vi "TurnScanParabolic2Components.vi"(0 "Start [s] AD raster":dbl=0.000225, 1 "TurnParameters":T1={"Turntime [s]"=4.500000000000001e-05, "Galvo cycle"=1e-05, "Pixeltime"=2.25e-06}, 2 "deltaPosition [m]":cluster{"x":dbl, "y":dbl}={"x"=-4.992779683200315e-05, "y"=-1.09458111857715e-05}, 4 "xPixel":i32=-99, 5 "speed [m/s]":cluster{"x":dbl, "y":dbl}={"x"=0.21752211986383552, "y"=0.04546254963512117}) -> (6 "Ende [s] AD+g raster":dbl=0.00027, 8 "ScanSteuerung":T2(array[cluster])=[{"Zeitpunkt [s]"=0.000225, "Wirkung"=enum."Inc", "Kanal"=enum."Image1X", "Wert (/s)"=-2315789.47368421}, {"Zeitpunkt [s]"=0.000225, "Wirkung"=enum."Rel", "Kanal"=enum."Image1Y", "Wert (/s)"=1.0}, {"Zeitpunkt [s]"=0.00023, "Wirkung"=enum."Abs", "Kanal"=enum."Digital", "Wert (/s)"=5.0}, {"Zeitpunkt [s]"=0.00023, "Wirkung"=enum."IncInc", "Kanal"=enum."GalvoX", "Wert (/s)"=-146143.4081327828}, {"Zeitpunkt [s]"=0.00023, "Wirkung"=enum."IncInc", "Kanal"=enum."GalvoY", "Wert (/s)"=-32321.565855881716}, {"Zeitpunkt [s]"=0.00025, "Wirkung"=enum."IncInc", "Kanal"=enum."GalvoX", "Wert (/s)"=146143.4081327828}, {"Zeitpunkt [s]"=0.00025, "Wirkung"=enum."IncInc", "Kanal"=enum."GalvoY", "Wert (/s)"=32321.565855881716}, {"Zeitpunkt [s]"=0.00026775000000000003, "Wirkung"=enum."Inc", "Kanal"=enum."Image1X", "Wert (/s)"=0.0}, {"Zeitpunkt [s]"=0.00027, "Wirkung"=enum."Abs", "Kanal"=enum."Digital", "Wert (/s)"=7.0}])   [LabVIEW 2011]
panel:
  out "t1":dbl=2e-05
  out "t0":dbl=2e-05
  out "x-y*floor(x/y)==galvoToo late":dbl=5.000000000000006e-06
  out "available galvo cycles":dbl=4.0
  # "For unidirectional!"
  # "ImageX is stopped before\ngalvos are still moving!"
  # "ImageX is stopped before\ngalvos are still moving!"
  # "Trigger Start Turn :101\nTrigger End Turn: 111"
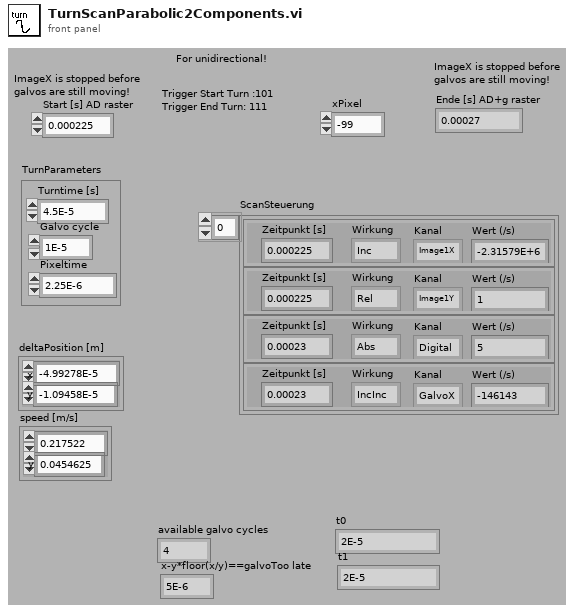
[diagram p1: front panel]
types:
  T1 = cluster{"Turntime [s]":dbl, "Galvo cycle":dbl, "Pixeltime":dbl}
  T2 = cluster{"Zeitpunkt [s]":dbl, "Wirkung":enum16{"Abs", "Rel", "Inc", "IncInc", "LoopStart", "LoopEnd"}, "Kanal":enum16{"Com", "AnalogConfig", "AnalogValue", "GalvoX", "GalvoY", "Galvo3", "Galvo4", "Digital", "Free", "Loop", "SMoveTime", "Image1X", "Image1Y", "Image2X", "Image2Y"}, "Wert (/s)":dbl}[]
  T3 = enum16{"Com", "AnalogConfig", "AnalogValue", "GalvoX", "GalvoY", "Galvo3", "Galvo4", "Digital", "Free", "Loop", "SMoveTime", "Image1X", "Image1Y", "Image2X", "Image2Y"}
  T4 = enum16{"Abs", "Rel", "Inc", "IncInc", "LoopStart", "LoopEnd"}
  T5 = cluster{"Start [s] AD raster":dbl, "Wirkung":enum16{"Abs", "Rel", "Inc", "IncInc", "LoopStart", "LoopEnd"}, "Kanal":enum16{"Com", "AnalogConfig", "AnalogValue", "GalvoX", "GalvoY", "Galvo3", "Galvo4", "Digital", "Free", "Loop", "SMoveTime", "Image1X", "Image1Y", "Image2X", "Image2Y"}, dbl}
  T6 = cluster{dbl, "Wirkung":enum16{"Abs", "Rel", "Inc", "IncInc", "LoopStart", "LoopEnd"}, "Kanal":enum16{"Com", "AnalogConfig", "AnalogValue", "GalvoX", "GalvoY", "Galvo3", "Galvo4", "Digital", "Free", "Loop", "SMoveTime", "Image1X", "Image1Y", "Image2X", "Image2Y"}, "y":dbl}
  T7 = cluster{dbl, "Wirkung":enum16{"Abs", "Rel", "Inc", "IncInc", "LoopStart", "LoopEnd"}, "Kanal":enum16{"Com", "AnalogConfig", "AnalogValue", "GalvoX", "GalvoY", "Galvo3", "Galvo4", "Digital", "Free", "Loop", "SMoveTime", "Image1X", "Image1Y", "Image2X", "Image2Y"}, "x":dbl}
  T8 = cluster{dbl, "Wirkung":enum16{"Abs", "Rel", "Inc", "IncInc", "LoopStart", "LoopEnd"}, "Kanal":enum16{"Com", "AnalogConfig", "AnalogValue", "GalvoX", "GalvoY", "Galvo3", "Galvo4", "Digital", "Free", "Loop", "SMoveTime", "Image1X", "Image1Y", "Image2X", "Image2Y"}, u8}
  T9 = cluster{"Start [s] AD raster":dbl, "Wirkung":enum16{"Abs", "Rel", "Inc", "IncInc", "LoopStart", "LoopEnd"}, "Kanal":enum16{"Com", "AnalogConfig", "AnalogValue", "GalvoX", "GalvoY", "Galvo3", "Galvo4", "Digital", "Free", "Loop", "SMoveTime", "Image1X", "Image1Y", "Image2X", "Image2Y"}, "y":dbl}[]
  T10 = cluster{"Start [s] AD raster":dbl, "Wirkung":enum16{"Abs", "Rel", "Inc", "IncInc", "LoopStart", "LoopEnd"}, "Kanal":enum16{"Com", "AnalogConfig", "AnalogValue", "GalvoX", "GalvoY", "Galvo3", "Galvo4", "Digital", "Free", "Loop", "SMoveTime", "Image1X", "Image1Y", "Image2X", "Image2Y"}, "xPixel":i32}
  T11 = cluster{dbl, "Wirkung":enum16{"Abs", "Rel", "Inc", "IncInc", "LoopStart", "LoopEnd"}, "Kanal":enum16{"Com", "AnalogConfig", "AnalogValue", "GalvoX", "GalvoY", "Galvo3", "Galvo4", "Digital", "Free", "Loop", "SMoveTime", "Image1X", "Image1Y", "Image2X", "Image2Y"}, dbl}
  T12 = typedef "ScanControl.ctl" = cluster{"Time [s]":dbl, "action":T13, "channel":T14, "value (/s)":dbl}[]
  T13 = typedef "ScanControl_Action.ctl" = enum16{"Abs", "Rel", "Inc", "IncInc", "LoopStart", "LoopEnd", "WaitTriggerRising"}
  T14 = typedef "ScanControl_Channel.ctl" = enum16{"Com", "AnalogConfig", "AnalogValue", "GalvoX", "GalvoY", "Galvo3", "Galvo4", "Digital", "Free", "Loop", "SMoveTime", "Image1X", "Image1Y", "Image2X", "Image2Y"}
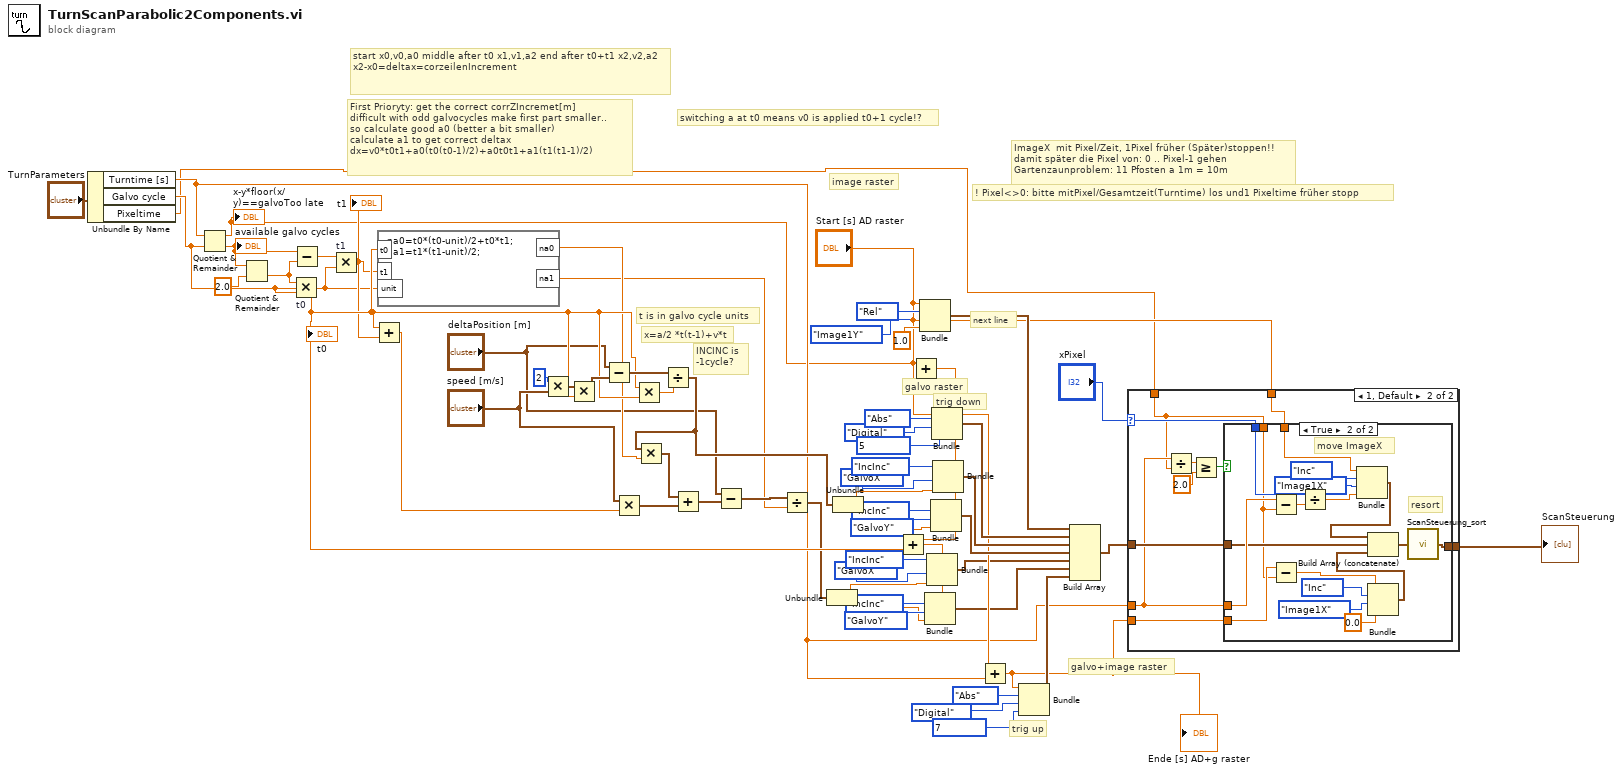
[diagram p0: block diagram]
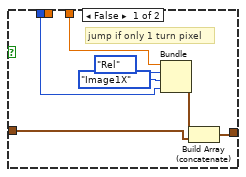
[diagram p3: hidden frame]
diagram:
  # "start x0,v0,a0 middle after t0 x1,v1,a2 end after t0+t1 x2,v2,a2\nx2-x0=deltax=corzeilenIncrement"
  # "First Prioryty: get the correct corrZIncremet[m]\ndifficult with odd galvocycles make first part smaller..\nso calculate good a0 (better a bit smaller)\ncalculate a1 to get correct deltax\ndx=v0*t0t1+a0(t0(t0-1)/2)+a0t0t1+a1(t1(t1-1)/2)"
  # "switching a at t0 means v0 is applied t0+1 cycle!?"
  # "t is in galvo cycle units"
  # "x=a/2 *t(t-1)+v*t"
  # "INCINC is\n-1cycle?"
  # "ImageX  mit Pixel/Zeit, 1Pixel früher (Später)stoppen!!\ndamit später die Pixel von: 0 .. Pixel-1 gehen\nGartenzaunproblem: 11 Pfosten a 1m = 10m"
  # "galvo+image raster"
  # "image raster"
  # "galvo raster"
  # "! Pixel<>0: bitte mitPixel/Gesamtzeit(Turntime) los und1 Pixeltime früher stopp"
  # "next line"
  # "trig up"
  # "trig down"
  n1 = Unbundle By Name("TurnParameters") -> ("Turntime [s]"=w4:dbl, "Galvo cycle"=w3:dbl, "Pixeltime"=w1:dbl)
  n2 = Quotient & Remainder(x=w4, y=w3) -> (x-y*floor(x/y)=w2:dbl, floor(x/y)=w35:dbl)
  "available galvo cycles" <- w35
  "x-y*floor(x/y)==galvoToo late" <- w2
  n3 = Quotient & Remainder(x=w35, y=2.0) -> (floor(x/y)=w34:dbl)  [unwired: 1 out]
  n4 = Multiply "t0"(x=w34, y=w3) -> (x*y=w16:dbl)
  "t0" <- w16
  n5 = Subtract(x=w35, y=w34) -> (x-y=w33:dbl)
  n6 = Multiply "t1"(x=w33, y=w3) -> (x*y=w15:dbl)
  "t1" <- w15
  n7 = Add(x=w16, y=w15) -> (x+y=w18:dbl)
  n8 = formula code="na0=t0*(t0-unit)/2+t0*t1;\nna1=t1*(t1-unit)/2;"("t0"=w16, "t1"=w15, "unit"=w3) -> ("na0"=w13:dbl, "na1"=w9:dbl)
  n9 = Multiply(x=2, y="speed [m/s]") -> (x*y=w21:cluster{"x":dbl, "y":dbl})
  n10 = Multiply(x=w21, y=w16) -> (x*y=w22:cluster{"x":dbl, "y":dbl})
  n11 = Subtract(x="deltaPosition [m]", y=w22) -> (x-y=w19:cluster{"x":dbl, "y":dbl})
  n12 = Multiply(x="speed [m/s]", y=w18) -> (x*y=w12:cluster{"x":dbl, "y":dbl})
  n13 = Multiply(x=w16, y=w16) -> (x*y=w37:dbl)
  n14 = Divide(x=w19, y=w37) -> (x/y=w14:cluster{"x":dbl, "y":dbl})
  n15 = Multiply(x=w14, y=w13) -> (x*y=w11:cluster{"x":dbl, "y":dbl})
  n16 = Add(x=w11, y=w12) -> (x+y=w7:cluster{"x":dbl, "y":dbl})
  n17 = Subtract(x="deltaPosition [m]", y=w7) -> (x-y=w10:cluster{"x":dbl, "y":dbl})
  n18 = Divide(x=w10, y=w9) -> (x/y=w8:cluster{"x":dbl, "y":dbl})
  n19 = Unbundle(w8) -> ("x"=w30:dbl, "y"=w23:dbl)
  n20 = Unbundle(w14) -> ("x"=w60:dbl, "y"=w59:dbl)
  n21 = Add(x="Start [s] AD raster", y=w2) -> (x+y=w24:dbl)
  n22 = Add(x=w24, y=w16) -> (x+y=w25:dbl)
  n23 = Bundle("Start [s] AD raster"="Start [s] AD raster", "Wirkung"=T4."Rel", "Kanal"=T3."Image1Y", 1.0) -> (w48:T5)  [unwired: 1 out]
  n24 = Bundle(w25, "Wirkung"=T4."IncInc", "Kanal"=T3."GalvoY", "y"=w23) -> (w26:T6)  [unwired: 1 out]
  n25 = Bundle(w25, "Wirkung"=T4."IncInc", "Kanal"=T3."GalvoX", "x"=w30) -> (w27:T7)  [unwired: 1 out]
  n26 = Bundle(w24, "Wirkung"=T4."IncInc", "Kanal"=T3."GalvoY", "y"=w59) -> (w55:T6)  [unwired: 1 out]
  n27 = Bundle(w24, "Wirkung"=T4."Abs", "Kanal"=T3."Digital", u8 5) -> (w49:T8)  [unwired: 1 out]
  n28 = Bundle(w24, "Wirkung"=T4."IncInc", "Kanal"=T3."GalvoX", "x"=w60) -> (w56:T7)  [unwired: 1 out]
  n29 = Add(x="Start [s] AD raster", y=w4) -> (x+y=w43:dbl)
  "Ende [s] AD+g raster" <- w43
  n30 = Bundle(w43, "Wirkung"=T4."Abs", "Kanal"=T3."Digital", u8 7) -> (w50:T8)  [unwired: 1 out]
  n31 = Build Array(w48, w49, w56, w55, w27, w26, w50) -> (w47:T9)
  n32 = case shown="1, Default" "xPixel" {
    selector: "xPixel" -> [_ w69]
    tunnel: w47 -> [w63 w72]
    tunnel: [w63 w71] -> w46
    tunnel: w4 -> [_ w68]
    tunnel: "Start [s] AD raster" -> [_ w73]
    tunnel: w43 -> [_ w70]
    tunnel: w1 -> [_ w67]
    frame 0 {
      # "no imageX movement"
    }
    frame 1, Default {
      n33 = Divide(x=w68, y=w67) -> (x/y=w66:dbl)
      n34 = Greater Or Equal?(x=w66, y=2.0) -> (x >= y?=w64:bool)
      n35 = case shown="True" w64 {
        tunnel: w68 -> [_ w97]
        tunnel: w73 -> [w74 w96]
        tunnel: w72 -> [w77 w94]
        tunnel: [w76 w89] -> w71
        tunnel: w70 -> [_ w88]
        tunnel: w69 -> [w75 w86]
        tunnel: w67 -> [_ w81]
        frame False {
          # "jump if only 1 turn pixel"
          n36 = Bundle("Start [s] AD raster"=w74, "Wirkung"=T4."Rel", "Kanal"=T3."Image1X", "xPixel"=w75) -> (w78:T10)  [unwired: 1 out]
          n37 = Build Array (concatenate)(w78, w77) -> (w76:T9)
        }
        frame True {
          # "move ImageX"
          # "resort"
          n38 = Subtract(x=w97, y=w81) -> (x-y=w85:dbl)
          n39 = Subtract(x=w88, y=w81) -> (x-y=w87:dbl)
          n40 = Divide(x=w86, y=w85) -> (x/y=w95:dbl)
          n41 = Bundle("Start [s] AD raster"=w96, "Wirkung"=T4."Inc", "Kanal"=T3."Image1X", w95) -> (w93:T5)  [unwired: 1 out]
          n42 = Bundle(w87, "Wirkung"=T4."Inc", "Kanal"=T3."Image1X", 0.0) -> (w90:T11)  [unwired: 1 out]
          n43 = Build Array (concatenate)(w93, w94, w90) -> (w82:T9)
          n44 = call "ScanSteuerung_sort.vi"("ScanSteuerung"=w82) -> ("ScanSteuerung"=w89:T12)
        }
      }
    }
  }
  "ScanSteuerung" <- w46
